vi "qVER.vi"(0 "System no.":i32=1 min=1 max=4 step=1, 5 "error in":errorcluster) -> (14 "Firmware version":string, 19 "error out":errorcluster)   [LabVIEW 2026]
doc: "GCS 3.0\n=====\n\nVER? (Get Version Information)\n\nDescription\nQueries the versions of the firmware and other components, such as driver and libraries.\n\nFormat\nVER?\n\nArguments\nnone\n\nResponse\nOutput format:\nThe Version Information block consists of at least the following fields:\n- HW-Matchcode Match code of the hardware\n- SN-Number Serial number of the hardware\n- Device-Type Type of firmware. Possible values:\n- FPGA-FW FPGA\n- CPU-FW x86 processor\n- DSP-FW Digital signal processor\n- MC-FW Other microcontroller\n- APP Main firmware for the hardware. This information must be available for every \nhardware component in a modular controller.\n- UMF Version of the UMF library. The UMF library contains amongst other things the \nGCS interpreter. For modular controllers, this information must be available for the \nmain hardware, but not for subordinate hardware components.\n- BL Bootloader\nIf there are several identical type designations within a controller, these are \nincremented: _1, _2, ...\n- 4-Digit Version Version information in the format <major version number>.<minor \nversion number>.<revision number>.<build number>\nThe Version Information block also contains the following fields if the current user command \nlevel is >= Developer:\n- Git-Hash Brief information on the Git revision\nExample\n>>ver?\n<<#Version Information: <HW-Matchcode> <SN-Number> <DeviceType> <4-Digit Version>\n<<UMF-DEMO 0000000000 APP 0.15.5.0\n<<UMF-DEMO 0000000000 UMF 0.15.5.0\n<<#END Version Information\n\nNotes\nThe *IDN? command (p. 7) queries the device identification string of the controller.\n\nUser command level\nUSR\n\n\nGCS 2.0\n=====\n\nReturns firmware string. \n\nC-867:"
panel:
  # "VER? (Get Version Information)\n\nQueries the versions of the firmware and other components, such as driver and libraries."
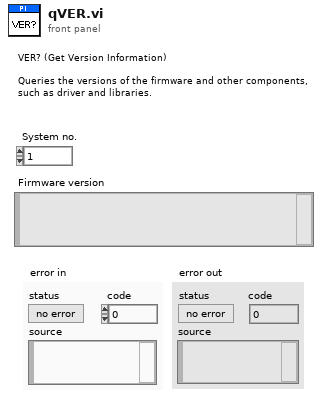
[diagram p1: front panel]
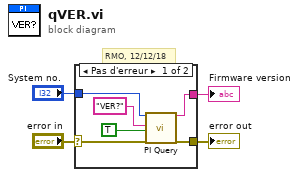
[diagram p0: block diagram]
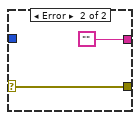
[diagram p2: hidden frame]
diagram:
  # "RMO, 12/12/18"
  n1 = case shown="Pas d'erreur" "error in" {
    selector: "error in" -> [w7 w12]
    tunnel: [w5 ""] -> w4
    tunnel: [w6 w12] -> w3
    tunnel: "System no." -> [w8 _]
    frame No Error {
      n2 = call "PI Query.vi"("System no."=w8, "String to send"="VER?" ("String to Send"), "Attach termination char.?"=TRUE ("Attach Linefeed?"), "error in"=w7) -> ("String read"=w5:string, "error out"=w6:errorcluster)  [unwired: 3 in, 11 out]
    }
    frame Error {
    }
  }
  "Firmware version" <- w4
  "error out" <- w3
